vi "Boiler room.vi"() -> ()   [LabVIEW 2023]
panel:
  out "Numeric":dbl
  in  "Heater":dbl(knob) min=0.0 max=2.0 step=1.0 scale=0.0..2.0
  in  "stop":bool
  out "Thermometer":dbl(slide) scale=0.0..100.0
  in  "min temp":dbl=20.0
  in  "max temp":dbl=80.0
  in  "Automatic / Manual":bool
  out "AC":bool
  out "Heater":bool
  # "OFF"
  # "AC"
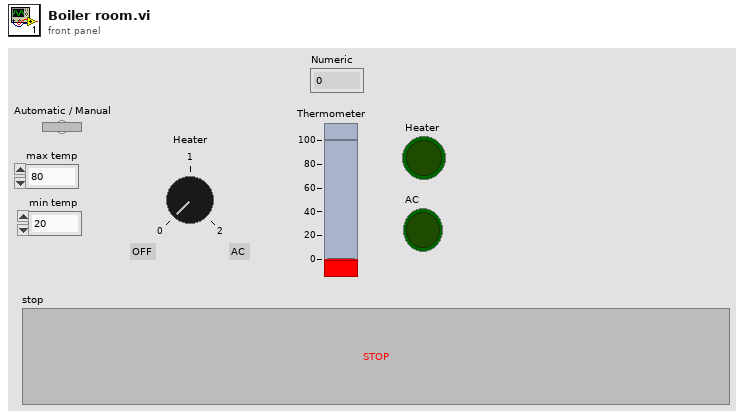
[diagram p1: front panel]
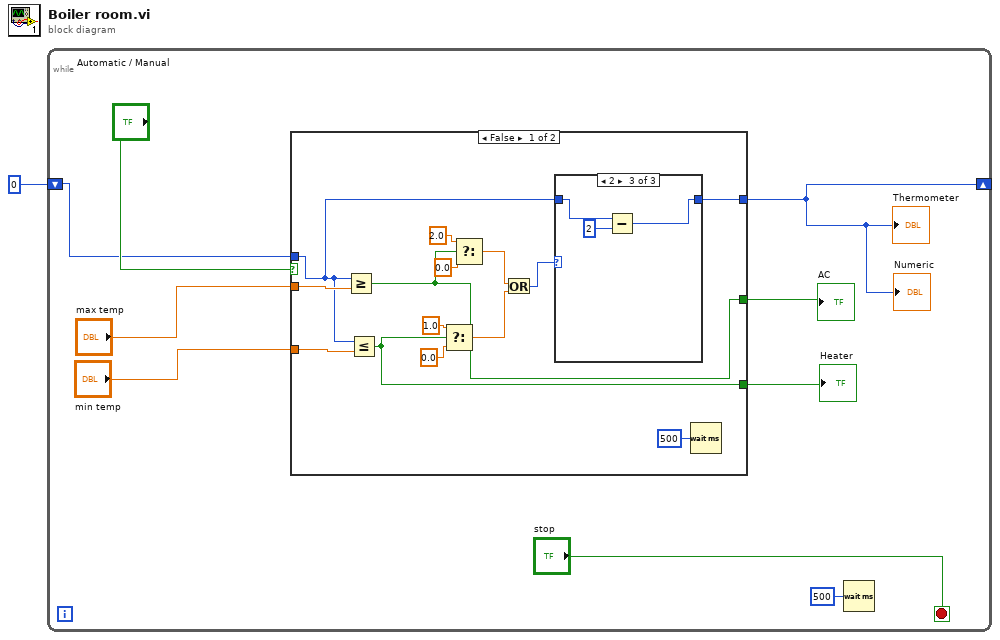
[diagram p0: block diagram]
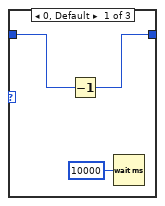
[diagram p2: hidden frame]
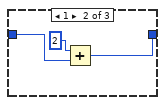
[diagram p3: hidden frame]
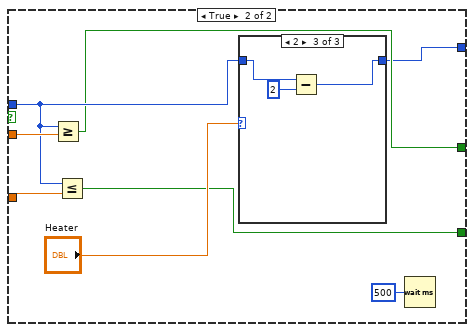
[diagram p4: hidden frame]
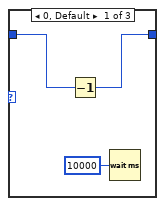
[diagram p5: hidden frame]
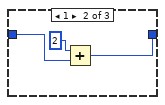
[diagram p6: hidden frame]
diagram:
  n1 = while {
    shift-right: [w2] -> _
    shift-left: 0 -> [w5]
    stop <- "stop" stop-if-true
    n2 = case shown="False" "Automatic / Manual" {
      tunnel: [w22 w36] -> w9
      tunnel: [w17 w37] -> w8
      tunnel: w5 -> [w13 w38]
      tunnel: "max temp" -> [w24 w40]
      tunnel: "min temp" -> [w23 w39]
      tunnel: [w12 w34] -> w2
      frame False {
        n3 = Greater Or Equal?(x=w13, y=w24) -> (x >= y?=w22:bool)
        n4 = Less Or Equal?(x=w13, y=w23) -> (x <= y?=w17:bool)
        n5 = Select(t=1.0, s=w17, f=0.0) -> (s? t:f=w16:dbl)
        n6 = Select(t=2.0, s=w22, f=0.0) -> (s? t:f=w15:dbl)
        n7 = Or(x=w15, y=w16) -> (x .or. y?=w14:i32)
        n8 = case shown="2" w14 {
          tunnel: w13 -> [w27 w30 w33]
          tunnel: [w26 w29 w32] -> w12
          frame 0, Default {
            n9 = Decrement(x=w27) -> (x-1=w26:i32)
            n10 = Wait (ms)(milliseconds to wait=u32 10000) -> ()  [unwired: 1 out]
          }
          frame 1 {
            n11 = Add(x=2, y=w30) -> (x+y=w29:i32)
          }
          frame 2 {
            n12 = Subtract(x=w33, y=2) -> (x-y=w32:i32)
          }
        }
        n13 = Wait (ms)(milliseconds to wait=u32 500) -> ()  [unwired: 1 out]
      }
      frame True {
        n14 = Greater Or Equal?(x=w38, y=w40) -> (x >= y?=w36:bool)
        n15 = Less Or Equal?(x=w38, y=w39) -> (x <= y?=w37:bool)
        n16 = case shown="2" "Heater" {
          tunnel: w38 -> [w44 w47 w50]
          tunnel: [w43 w46 w49] -> w34
          frame 0, Default {
            n17 = Decrement(x=w44) -> (x-1=w43:i32)
            n18 = Wait (ms)(milliseconds to wait=u32 10000) -> ()  [unwired: 1 out]
          }
          frame 1 {
            n19 = Add(x=2, y=w47) -> (x+y=w46:i32)
          }
          frame 2 {
            n20 = Subtract(x=w50, y=2) -> (x-y=w49:i32)
          }
        }
        n21 = Wait (ms)(milliseconds to wait=u32 500) -> ()  [unwired: 1 out]
      }
    }
    "Heater" <- w8
    "AC" <- w9
    "Thermometer" <- w2
    "Numeric" <- w2
    n22 = Wait (ms)(milliseconds to wait=u32 500) -> ()  [unwired: 1 out]
  }
